vi "Vacuum Test - Step 5.vi"(7 "Step":i32, 8 "error in":errorcluster, 9 "Test Results":T9, 10 "Oil In":T1, 11 "Test Configuration":T2) -> (0 "error out":errorcluster, 1 "Test Results Out":T9, 2 "Oil Out":T1, 3 "Test Configuration Out":T2)   [LabVIEW 2015]
uses:
  Controls/Test Results.ctl
  Controls/Step Result.ctl
  Controls/Startup Test.ctl
  Controls/Test Information.ctl
  Controls/Vacuum Test.ctl
  Controls/Test Timing.ctl
  Controls/Vaccum Thresholds.ctl
  Controls/Helium Test.ctl
  Controls/Helium Thresholds.ctl
  Controls/Startup Thresholds.ctl
  CAN Communication/Oil/Typedefs/Session Handle.ctl
  CAN Communication/Oil/Oil.lvclass
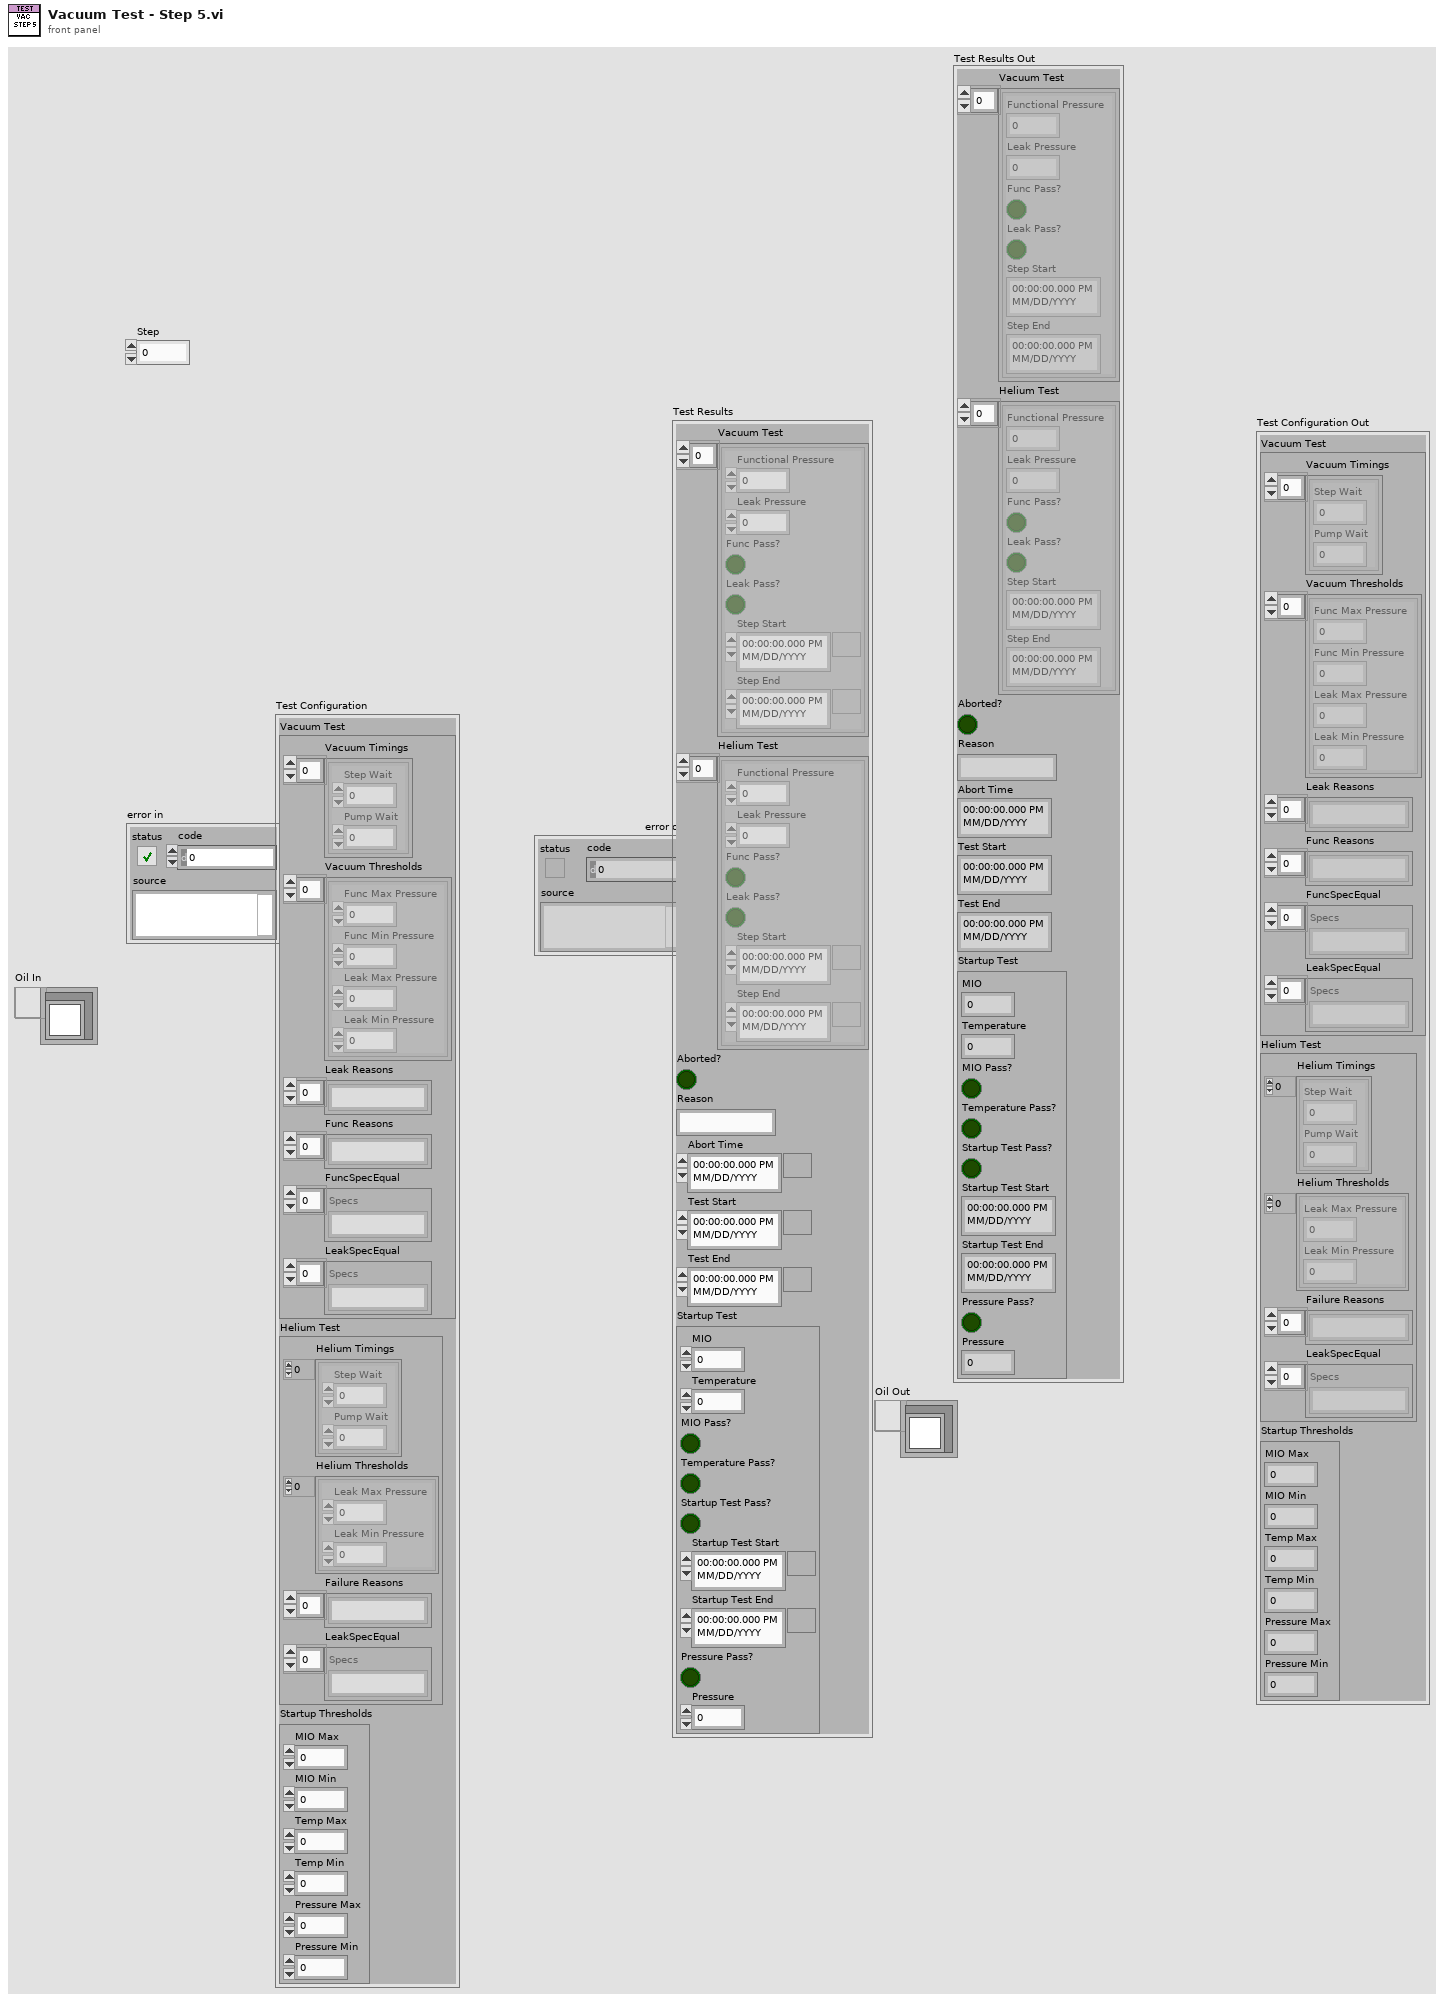
[diagram p1: front panel]
types:
  T1 = typedef "Oil.lvclass/Session Handle.ctl" = refnum<data-value>
  T2 = typedef "Test Information.ctl" = cluster{"Vacuum Test":T3, "Helium Test":T6, "Startup Thresholds":T8}
  T3 = typedef "Vacuum Test.ctl" = cluster{"Vacuum Timings":T4[], "Vacuum Thresholds":T5[], "Leak Reasons":string[], "Func Reasons":string[], "FuncSpecEqual":string[], "LeakSpecEqual":string[]}
  T4 = typedef "Test Timing.ctl" = cluster{"Step Wait":dbl, "Pump Wait":dbl}
  T5 = typedef "Vaccum Thresholds.ctl" = cluster{"Func Max Pressure":dbl, "Func Min Pressure":dbl, "Leak Max Pressure":dbl, "Leak Min Pressure":dbl}
  T6 = typedef "Helium Test.ctl" = cluster{"Helium Timings":T4[], "Helium Thresholds":T7[], "Failure Reasons":string[], "LeakSpecEqual":string[]}
  T7 = typedef "Helium Thresholds.ctl" = cluster{"Leak Max Pressure":dbl, "Leak Min Pressure":dbl}
  T8 = typedef "Startup Thresholds.ctl" = cluster{"MIO Max":dbl, "MIO Min":dbl, "Temp Max":dbl, "Temp Min":dbl, "Pressure Max":dbl, "Pressure Min":dbl}
  T9 = typedef "Test Results.ctl" = cluster{"Vacuum Test":T10[], "Helium Test":T10[], "Aborted?":bool, "Reason":string, "Abort Time":timestamp, "Test Start":timestamp, "Test End":timestamp, "Startup Test":T11}
  T10 = typedef "Step Result.ctl" = cluster{"Functional Pressure":dbl, "Leak Pressure":dbl, "Func Pass?":bool, "Leak Pass?":bool, "Step Start":timestamp, "Step End":timestamp}
  T11 = typedef "Startup Test.ctl" = cluster{"MIO":dbl, "Temperature":dbl, "MIO Pass?":bool, "Temperature Pass?":bool, "Startup Test Pass?":bool, "Startup Test Start":timestamp, "Startup Test End":timestamp, "Pressure Pass?":bool, "Pressure":dbl}
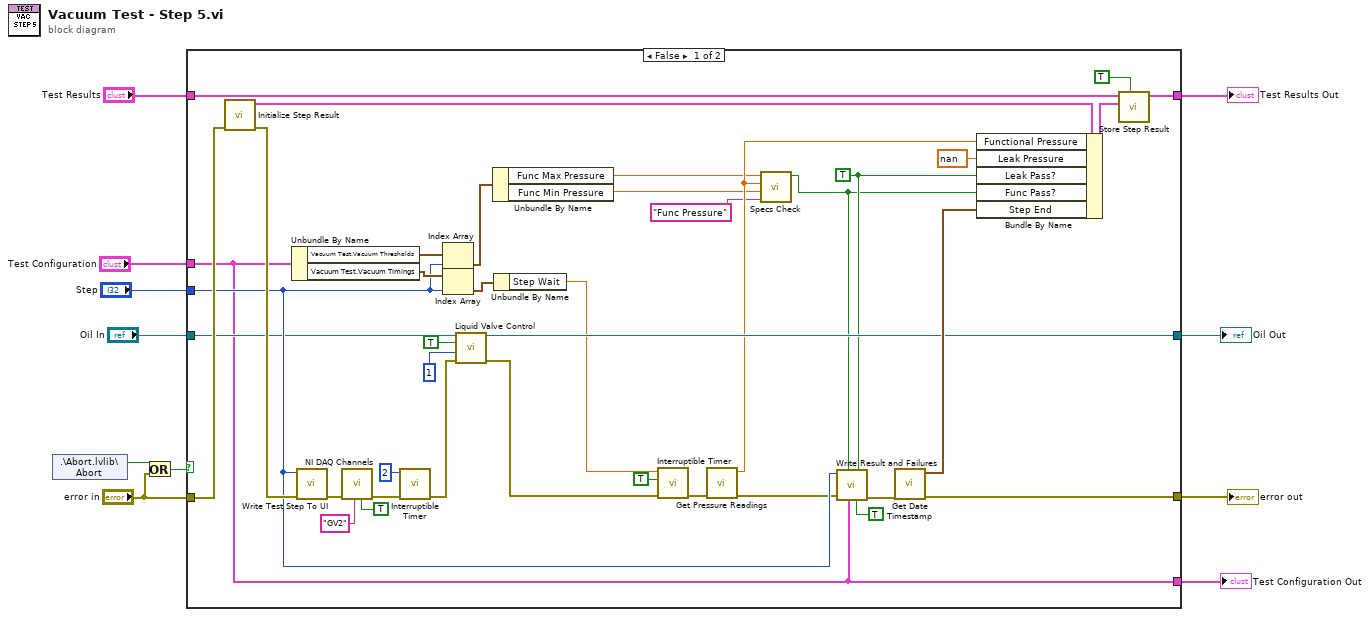
[diagram p0: block diagram]
diagram:
  n1 = shared-variable ".\\Abort.lvlib\\Abort"() -> (w10:bool)  [unwired: 1 in, 1 out]
  n2 = Or(x=w10, y="error in") -> (x .or. y?=w9:bool)
  n3 = case shown="False" w9 {
    tunnel: "error in" -> [w50 w53]
    tunnel: "Test Results" -> [w47 w54]
    tunnel: [w48 w54] -> w8
    tunnel: [w35 w53] -> w7
    tunnel: "Test Configuration" -> [w19 w52]
    tunnel: "Step" -> [w38 _]
    tunnel: [w19 w52] -> w3
    tunnel: [w30 w51] -> w1
    tunnel: "Oil In" -> [w31 w51]
    frame False {
      w21 = TRUE ("Leak Pass?")
      n4 = call "Initialize Step Result.vi"("error in (no error)"=w50) -> ("error out"=w49:errorcluster, "New Step Result"=w46:T10)  [unwired: 8 in, 1 out]
      n5 = Unbundle By Name(w19) -> ("Vacuum Test.Vacuum Thresholds"=w43:T5[], "Vacuum Test.Vacuum Timings"=w42:T4[])
      n6 = call "Write Test Step To UI.vi"("error in (no error)"=w49, "Step"=w38) -> ("error out"=w32:errorcluster)  [unwired: 9 in]
      n7 = call "NI DAQ Channels.vi"("Control"=TRUE ("State"), "Channel"="GV2", "error in (no error)"=w32) -> ("error out"=w33:errorcluster)  [unwired: 7 in, 1 out]
      n8 = call "Interruptible Timer.vi"("error in (no error)"=w33, "Wait (s)"=2) -> ("error out"=w29:errorcluster)  [unwired: 7 in, 2 out]
      n9 = Index Array(array=w43, index=w38) -> (element=w39:T5)
      n10 = Index Array(array=w42, index=w38) -> (element=w41:T4)
      n11 = call "Liquid Valve Control.vi"("Session Handle in"=w31, "On?"=TRUE, "Valve"=1, "error in (no error)"=w29) -> ("Session Handle out"=w30:T1, "error out"=w26:errorcluster)  [unwired: 8 in, 2 out]
      n12 = Unbundle By Name(w39) -> ("Func Max Pressure"=w15:dbl, "Func Min Pressure"=w14:dbl)
      n13 = Unbundle By Name(w41) -> ("Step Wait"=w25:dbl)
      n14 = call "Interruptible Timer.vi"("error in (no error)"=w26, "Update UI?"=TRUE, "Wait (s)"=w25) -> ("error out"=w23:errorcluster)  [unwired: 6 in, 2 out]
      n15 = call "Get Pressure Readings.vi"("error in (no error)"=w23) -> ("error out"=w22:errorcluster, "NI-DAQ Pressure"=w16:dbl)  [unwired: 7 in, 2 out]
      n16 = call "Specs Check.vi"("parameter"="Func Pressure", "lower limit"=w14, "x"=w16, "upper limit"=w15) -> ("In Range?"=w13:bool)  [unwired: 6 in, 1 out]
      n17 = call "Write Result and Failures.vi"("Vacuum?"=TRUE, "Leak"=w21, "Test Configuration"=w19, "Func"=w13, "error in (no error)"=w22, "Step"=w38) -> ("error out"=w36:errorcluster)  [unwired: 5 in]
      n18 = call "Get Date Timestamp.vi"("error in (no error)"=w36) -> ("error out"=w35:errorcluster, "current time"=w44:timestamp)  [unwired: 9 in]
      n19 = Bundle By Name(cluster=w46, "Functional Pressure"=w16, "Leak Pressure"=nan, "Leak Pass?"=w21, "Func Pass?"=w13, "Step End"=w44) -> (w45:T10)
      n20 = call "Store Step Result.vi"("Vacuum?"=TRUE, "Step Result"=w45, "Test Results In"=w47) -> ("Test Results Out"=w48:T9)  [unwired: 8 in]
    }
    frame True {
    }
  }
  "error out" <- w7
  "Test Results Out" <- w8
  "Test Configuration Out" <- w3
  "Oil Out" <- w1
